vi "Math-Truncated Exponential Distribution.vi"(0 "samples":i32, 5 "Min":dbl, 7 "Max":dbl, 9 "Lambda":dbl) -> (4 "Array":dbl[](array[numeric]))   [LabVIEW 2015]
uses:
  <vilib>/gmath/statdist.llb/Uniform Random.vi
  <vilib>/gmath/NI_Gmath.lvlib
  <vilib>/Analysis/NI_AALBase.lvlib
panel:
  out "Histogram":T1(graph)
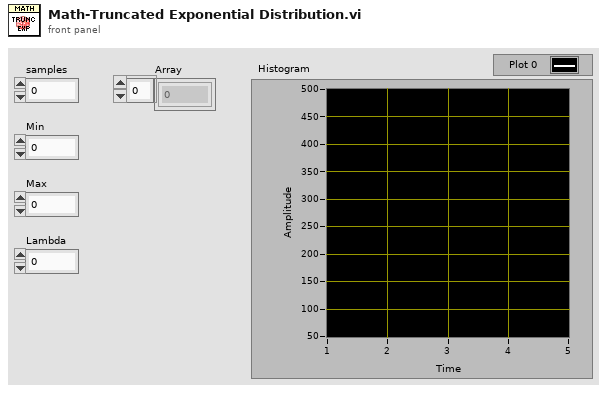
[diagram p1: front panel]
types:
  T1 = cluster{"X Values":dbl[], "Histogram: h(x)":i32[]}
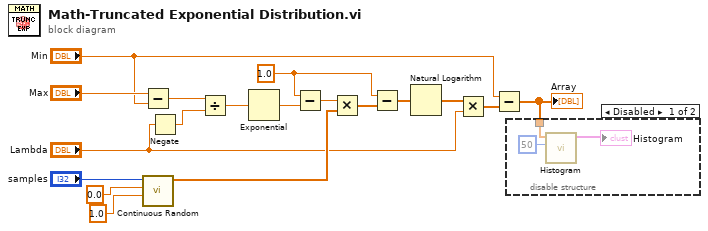
[diagram p0: block diagram]
diagram:
  w7 = 1.0
  n1 = Subtract(x="Max", y="Min") -> (x-y=w14:dbl)
  n2 = call-poly <vilib>:"Continuous Random.vi"("xmax"=1.0, "xmin"=0.0, "samples"="samples") -> ("uniform random data"=w9:dbl[])  [unwired: 7 in, 1 out]
  n3 = Negate(x="Lambda") -> (-x=w13:dbl)
  n4 = Divide(x=w14, y=w13) -> (x/y=w12:dbl)
  n5 = Exponential(1:w12) -> (0:w11:dbl)
  n6 = Subtract(x=w7, y=w11) -> (x-y=w10:dbl)
  n7 = Multiply(x=w10, y=w9) -> (x*y=w8:dbl[])
  n8 = Subtract(x=w7, y=w8) -> (x-y=w6:dbl[])
  n9 = Natural Logarithm(1:w6) -> (0:w5:dbl[])
  n10 = Multiply(x=w5, y="Lambda") -> (x*y=w3:dbl[])
  n11 = Subtract(x="Min", y=w3) -> (x-y=w1:dbl[])
  "Array" <- w1
  n12 = disable-structure shown="Disabled" {
    disable-tunnel: w1 -> [w21 _]
    frame Disabled {
      n13 = call <vilib>:"Histogram.vi"("intervals"=50, "X"=w21) -> ("Histogram Graph"=→"Histogram":T1)  [unwired: 6 in, 3 out]
    }
    frame Enabled {
    }
  }
